vi "hierarchical menu demo.vi"() -> ()   [LabVIEW 2010]
panel:
  out "selection":u32[](array[numeric])
  in  "set points":string[](array[string])=["setpoint 1", "setpoint 2", "setpoints 3", "set point 4", "set point 5", "set point 6"]
  in  "stop":bool
  in  "sensors":string[](array[string])=["sensor 1", "sensor 2", "sensor 3"]
  in  "Ring 2":u16(ring) items=["sensor 1", "sensor 2", "sensor 3"]
  in  "Ring":u16(ring) items=["elapsed time in current state", "sensor value", "Set point"]
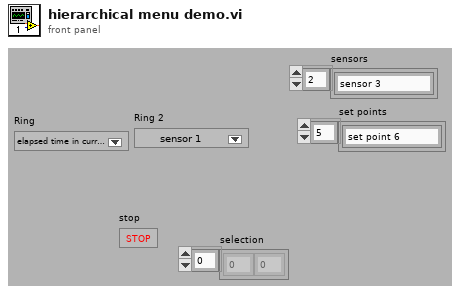
[diagram p1: front panel]
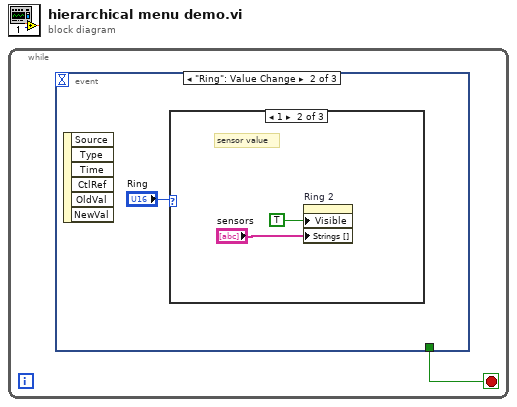
[diagram p0: block diagram]
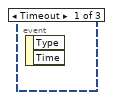
[diagram p2: hidden frame]
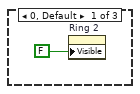
[diagram p3: hidden frame]
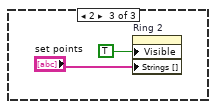
[diagram p4: hidden frame]
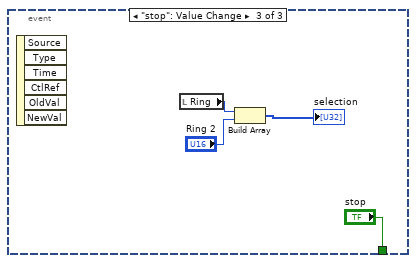
[diagram p5: hidden frame]
diagram:
  n1 = while {
    stop <- w1 stop-if-true
    n2 = event shown="[1] \"Ring\": Value Change" {
      selector: _ -> [_ _ _]
      dyn-events: _ -> [_ _ _]
      timeout: _ -> [_ _ _]
      tunnel: [_ _ "stop"] -> w1
      event Timeout {
        n3 = event-data() -> ()  [unwired: 1 in, 2 out]
      }
      event "Ring": Value Change {
        n4 = event-data() -> ()  [unwired: 1 in, 6 out]
        n5 = case shown="1" "Ring" {
          frame 0, Default {
            n6 = property on="Ring 2" class="Ring (strict)"("Visible"=FALSE) -> ()  [unwired: 2 in, 2 out]
          }
          frame 1 {
            # "sensor value"
            n7 = property on="Ring 2" class="Ring (strict)"("Visible"=TRUE, "Strings []"="sensors") -> ()  [unwired: 2 in, 2 out]
          }
          frame 2 {
            n8 = property on="Ring 2" class="Ring (strict)"("Visible"=TRUE, "Strings []"="set points") -> ()  [unwired: 2 in, 2 out]
          }
        }
      }
      event "stop": Value Change {
        n9 = event-data() -> ()  [unwired: 1 in, 6 out]
        n10 = local read "Ring"() -> (w10:u16)
        n11 = Build Array(w10, "Ring 2") -> (→"selection":u16[])
      }
    }
  }
